vi "ADIS16470 Scale Data.vi"(3 "TimeStamp":u32, 5 "Data In":u8[](array[numeric])) -> (1 "Scaled Data Out":dbl[](array[numeric]))   [LabVIEW 2019]
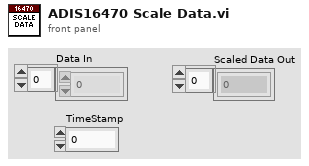
[diagram p1: front panel]
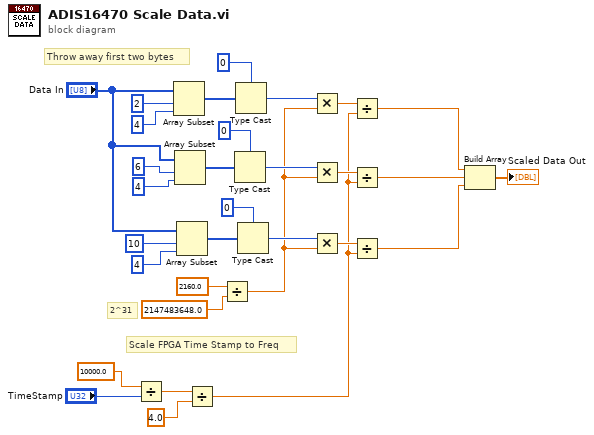
[diagram p0: block diagram]
diagram:
  # "Scale FPGA Time Stamp to Freq"
  # "2^31"
  # "Throw away first two bytes"
  n1 = Divide(x=10000.0, y="TimeStamp") -> (x/y=w3:dbl)
  n2 = Array Subset(array="Data In", index=2, length=4) -> (w24:u8[])
  n3 = Array Subset(array="Data In", index=6, length=4 ("index")) -> (w22:u8[])
  n4 = Array Subset(array="Data In", index=10, length=4) -> (w23:u8[])
  n5 = Divide(x=w3, y=4.0) -> (x/y=w1:dbl)
  n6 = Divide(x=2160.0, y=2147483648.0) -> (x/y=w12:dbl)
  n7 = Type Cast(type=0, x=w22) -> (*(type *) &x=w16:i32)
  n8 = Type Cast(type=0, x=w24) -> (*(type *) &x=w18:i32)
  n9 = Type Cast(type=0, x=w23) -> (*(type *) &x=w17:i32)
  n10 = Multiply(x=w18, y=w12) -> (x*y=w11:dbl)
  n11 = Multiply(x=w16, y=w12) -> (x*y=w10:dbl)
  n12 = Multiply(x=w17, y=w12) -> (x*y=w9:dbl)
  n13 = Divide(x=w11, y=w1) -> (x/y=w6:dbl)
  n14 = Divide(x=w10, y=w1) -> (x/y=w7:dbl)
  n15 = Divide(x=w9, y=w1) -> (x/y=w8:dbl)
  n16 = Build Array(w6, w7, w8) -> (→"Scaled Data Out":dbl[])
